vi "TrapProfile_ShouldFlipAcceleration.vi"(9 "goal TRAPEZOID_PROFILE_STATE":T1 {"Velocity" format="%16_6e"; "Position" format="%16_6e"}, 11 "Initial TRAPEZOID_PROFILE_STATE":T1 {"Velocity" format="%16_6e"; "Position" format="%16_6e"}) -> (3 "Flip":bool)   [LabVIEW 2019, in "Trajectory_Library.lvlib"]
doc: "DO NOT USE. THIS IS AN INTERNAL ONLY ROUTINE.\n \nReturns true if the profile inverted.\n \nThe profile is inverted if goal position is less than the initial position.\n \nInputs:\n - initial The initial state (usually the current state).\n - goal The desired state when the profile is complete.\n\nOutputs:\n - flip -- True if the profile is inverted."
uses:
  Trajectory_Library.lvlib
  TRAPEZOID_PROFILE_STATE.ctl
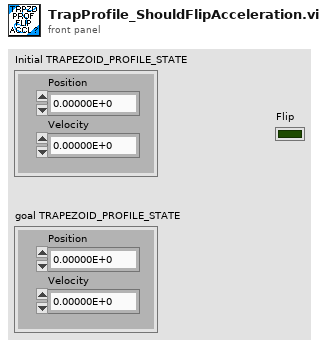
[diagram p1: front panel]
types:
  T1 = typedef "Trajectory_Library.lvlib/TRAPEZOID_PROFILE_STATE.ctl" = cluster{"Position":dbl, "Velocity":dbl}
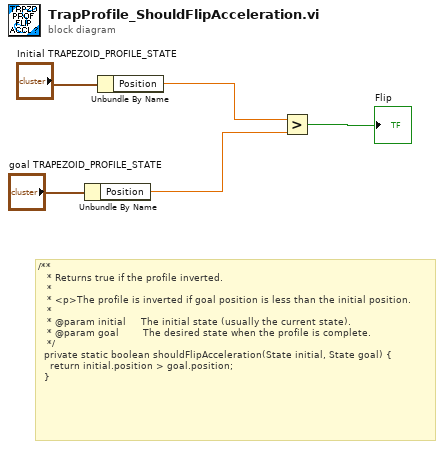
[diagram p0: block diagram]
diagram:
  # "/**\n   * Returns true if the profile inverted.\n   *\n   * <p>The profile is inverted if goal position is less than the initial position.\n   *\n   * @param initial     The initial state (usually the current state).\n   * @param goal        The desired state when the profile is complete.\n   */\n  private static boolean shouldFlipAcceleration(State initial, State goal) {\n    return initial.position > goal.position;\n  }"
  n1 = Unbundle By Name("goal TRAPEZOID_PROFILE_STATE") -> ("Position"=w2:dbl)
  n2 = Unbundle By Name("Initial TRAPEZOID_PROFILE_STATE") -> ("Position"=w3:dbl)
  n3 = Greater?(x=w3, y=w2) -> (0:→"Flip":bool)
